vi "Abort.vi"(6 "Message Queue":refnum<queue>, 8 "error in (no error)":errorcluster, 11 "Status":T1) -> (0 "error out":errorcluster, 3 "Status":T1)   [LabVIEW 2016]
doc: "This VI (called when the wash is aborted) will:\n- disable everything on the entry console\n- stop executing the current state\n- turn all wash indicators off\n- set the out of position indicator to red\n- set time remaining to 0.00\n- display an error dialog"
uses:
  Controls/Controller Status.ctl
  Architecture/Message Queue/Message Cluster.ctl
  Simulated Console/Controls/Button state.ctl
  Controls/Steps.ctl
  Controls/Stations.ctl
  Controls/Waiting States.ctl
  Architecture/Message Queue/Message Queue.lvlib
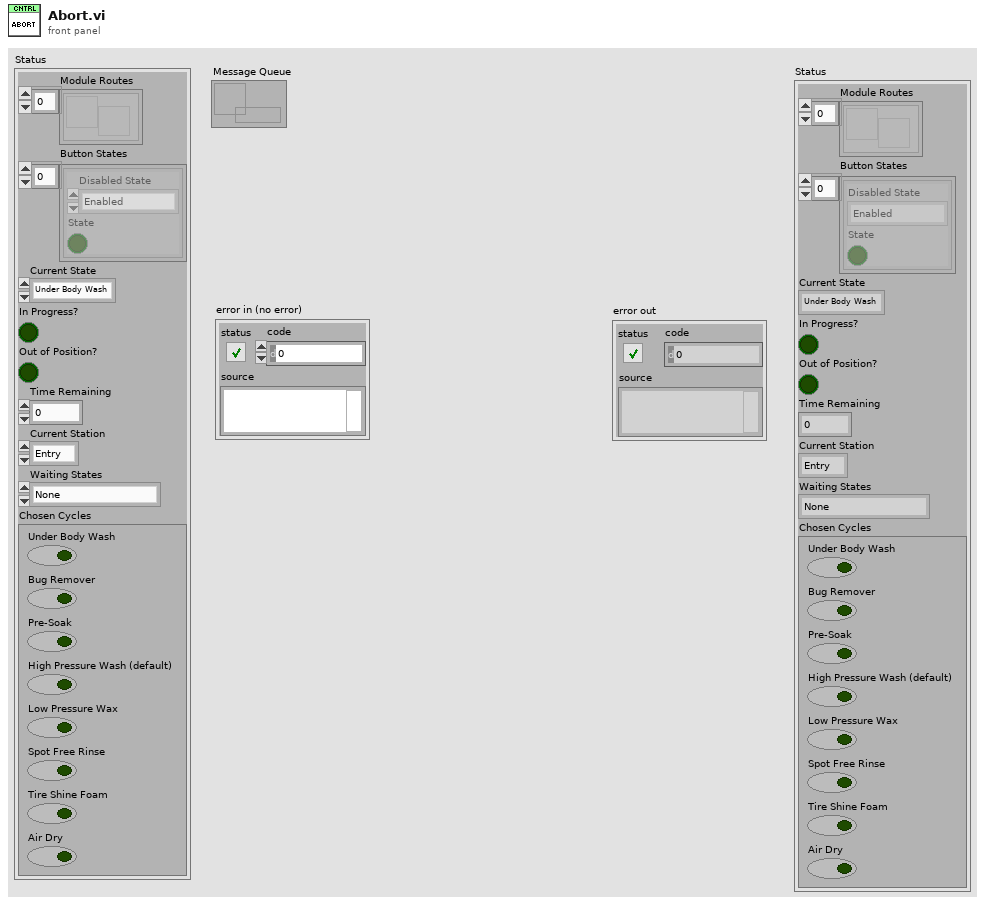
[diagram p1: front panel]
types:
  T1 = typedef "Controller Status.ctl" = cluster{"Module Routes":refnum<user-event>[], "Button States":T2[], "Current State":T3, "In Progress?":bool, "Out of Position?":bool, "Time Remaining":dbl, "Current Station":T4, "Waiting States":T5, "Chosen Cycles":cluster{"Under Body Wash":bool, "Bug Remover":bool, "Pre-Soak":bool, "High Pressure Wash (default)":bool, "Low Pressure Wax":bool, "Spot Free Rinse":bool, "Tire Shine Foam":bool, "Air Dry":bool}}
  T2 = typedef "Button state.ctl" = cluster{"Disabled State":enum8{"Enabled", "Disabled", "Disabled and Grayed Out"}, "State":bool}
  T3 = typedef "Steps.ctl" = enum16{"Under Body Wash", "Bug Remover", "Pre-Soak", "High Pressure Wash", "Low Pressure Wax", "Spot Free Rinse", "Tire Shine Foam", "Air Dry"}
  T4 = typedef "Stations.ctl" = enum16{"Entry", "Station 1", "Station 2", "Station 3", "Exit"}
  T5 = typedef "Waiting States.ctl" = enum16{"None", "for Start", "for Vehicle Position"}
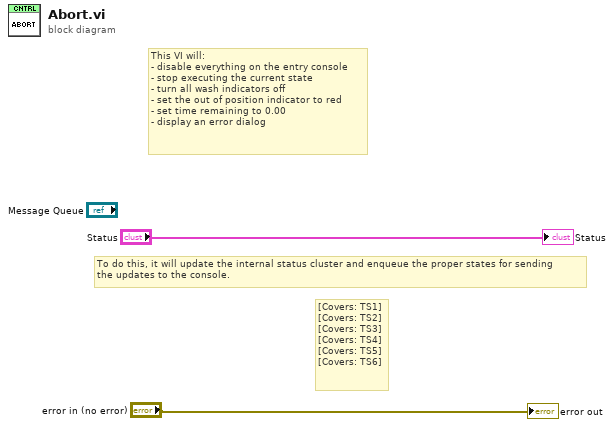
[diagram p0: block diagram]
diagram:
  # "To do this, it will update the internal status cluster and enqueue the proper states for sending\nthe updates to the console."
  # "[Covers: TS1]\n[Covers: TS2]\n[Covers: TS3]\n[Covers: TS4]\n[Covers: TS5]\n[Covers: TS6]"
  # "This VI will:\n- disable everything on the entry console\n- stop executing the current state\n- turn all wash indicators off\n- set the out of position indicator to red\n- set time remaining to 0.00\n- display an error dialog"
  "error out" <- "error in (no error)"
  "Status" <- "Status"
